vi "NN_Deploy.vi"(4 "Output Layer":cluster{"xgain 2":dbl[][], "xoffset 2":dbl[][]}, 5 "Input Layer":cluster{"xoffset":dbl[][], "xgain":dbl[][]}, 6 "Layer 2":T1, 7 "Layer 1":T2, 10 "Input":dbl[](array[numeric])) -> (2 "Output":dbl[](array[numeric]))   [LabVIEW 2018]
uses:
  <vilib>/Analysis/Matrix/Numeric/Conversions/Array To Matrix - RA2.vi
  <vilib>/Analysis/Matrix/Numeric/Multiply/Multiply - RM,RM.vi
  <vilib>/Analysis/Matrix/Numeric/Add/Add - RM,RM.vi
  <vilib>/Analysis/Matrix/Numeric/Conversions/Matrix To Array - RM.vi
  <vilib>/Analysis/Matrix/NI_Matrix.lvlib
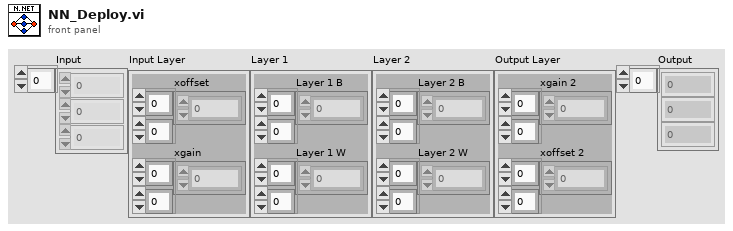
[diagram p1: front panel]
types:
  T1 = cluster{"Layer 2 B":dbl[][], "Layer 2 W":dbl[][]}
  T2 = cluster{"Layer 1 B":dbl[][], "Layer 1 W":dbl[][]}
  T3 = typedef "NI_Matrix.lvlib/RealMatrix.ctl" = dbl[][]
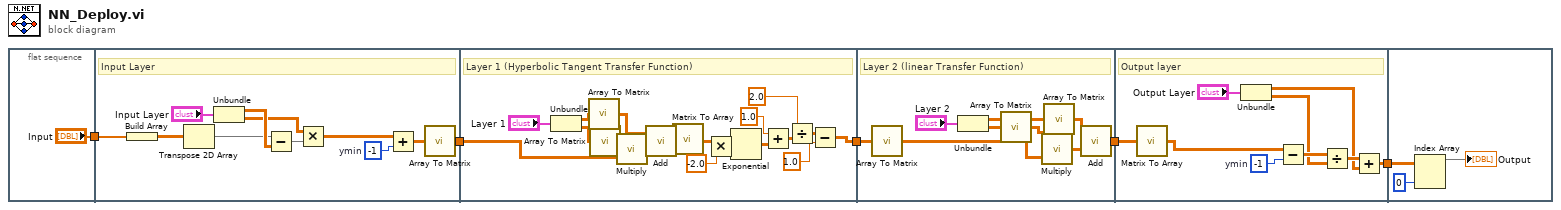
[diagram p0: block diagram]
diagram:
  n1 = flat-sequence {
    tunnel: ["Input"] -> w3
    tunnel: [w12] -> w5
    tunnel: w3 -> [w17]
    tunnel: w5 -> [w29]
    tunnel: [w21] -> w1
    tunnel: [w42] -> w4
    tunnel: w1 -> [w38]
    tunnel: w4 -> [w52]
    tunnel: [w50] -> w2
    tunnel: w2 -> [w56]
    frame #0 {
    }
    frame #1 {
      w14 = -1  # ymin
      # "Input Layer"
      n2 = Build Array(w17) -> (w10:dbl[][])
      n3 = Transpose 2D Array(2D array=w10) -> (transposed array=w7:dbl[][])
      n4 = Unbundle("Input Layer") -> ("xoffset"=w9:dbl[][], "xgain"=w8:dbl[][])
      n5 = Subtract(x=w7, y=w9) -> (x-y=w16:dbl[][])
      n6 = Multiply(x=w8, y=w16) -> (x*y=w15:dbl[][])
      n7 = Add(x=w15, y=w14) -> (x+y=w13:dbl[][])
      n8 = call-poly <vilib>:"Array To Matrix.vi"("Real 2D Array"=w13) -> ("Real Matrix"=w12:T3)
    }
    frame #2 {
      # "Layer 1 (Hyperbolic Tangent Transfer Function)"
      n9 = Unbundle("Layer 1") -> ("Layer 1 B"=w33:dbl[][], "Layer 1 W"=w31:dbl[][])
      n10 = call-poly <vilib>:"Array To Matrix.vi"("Real 2D Array"=w33) -> ("Real Matrix"=w32:T3)
      n11 = call-poly <vilib>:"Array To Matrix.vi"("Real 2D Array"=w31) -> ("Real Matrix"=w30:T3)
      n12 = call-poly <vilib>:"Multiply.vi"("Real Matrix B"=w29, "Real Matrix A"=w30) -> ("A * B"=w35:T3)
      n13 = call-poly <vilib>:"Add.vi"("Real Matrix B"=w35, "Real Matrix A"=w32) -> ("A + B"=w28:T3)
      n14 = call-poly <vilib>:"Matrix To Array.vi"("Real Matrix"=w28) -> ("Real 2D Array"=w26:dbl[][])
      n15 = Multiply(x=w26, y=-2.0) -> (x*y=w25:dbl[][])
      n16 = Exponential(1:w25) -> (0:w20:dbl[][])
      n17 = Add(x=1.0, y=w20) -> (x+y=w19:dbl[][])
      n18 = Divide(x=2.0, y=w19) -> (x/y=w23:dbl[][])
      n19 = Subtract(x=w23, y=1.0) -> (x-y=w21:dbl[][])
    }
    frame #3 {
      # "Layer 2 (linear Transfer Function)"
      n20 = call-poly <vilib>:"Array To Matrix.vi"("Real 2D Array"=w38) -> ("Real Matrix"=w36:T3)
      n21 = Unbundle("Layer 2") -> ("Layer 2 B"=w39:dbl[][], "Layer 2 W"=w40:dbl[][])
      n22 = call-poly <vilib>:"Array To Matrix.vi"("Real 2D Array"=w40) -> ("Real Matrix"=w37:T3)
      n23 = call-poly <vilib>:"Multiply.vi"("Real Matrix B"=w36, "Real Matrix A"=w37) -> ("A * B"=w44:T3)
      n24 = call-poly <vilib>:"Array To Matrix.vi"("Real 2D Array"=w39) -> ("Real Matrix"=w43:T3)
      n25 = call-poly <vilib>:"Add.vi"("Real Matrix B"=w44, "Real Matrix A"=w43) -> ("A + B"=w42:T3)
    }
    frame #4 {
      w51 = -1  # ymin
      # "Output layer"
      n26 = call-poly <vilib>:"Matrix To Array.vi"("Real Matrix"=w52) -> ("Real 2D Array"=w48:dbl[][])
      n27 = Unbundle("Output Layer") -> ("xgain 2"=w45:dbl[][], "xoffset 2"=w46:dbl[][])
      n28 = Subtract(x=w48, y=w51) -> (x-y=w47:dbl[][])
      n29 = Divide(x=w47, y=w46) -> (x/y=w53:dbl[][])
      n30 = Add(x=w53, y=w45) -> (x+y=w50:dbl[][])
    }
    frame #5 {
      n31 = Index Array(array=w56, index (col)=0 ("disabled index (col)")) -> (element=→"Output":dbl[])  [unwired: 1 in]
    }
  }
